vi "TreDadi.vi"() -> (1 "Dado_3":u32, 2 "Dado_2":u32, 3 "Dado_1":u32)   [LabVIEW 2013]
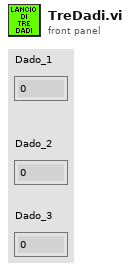
[diagram p1: front panel]
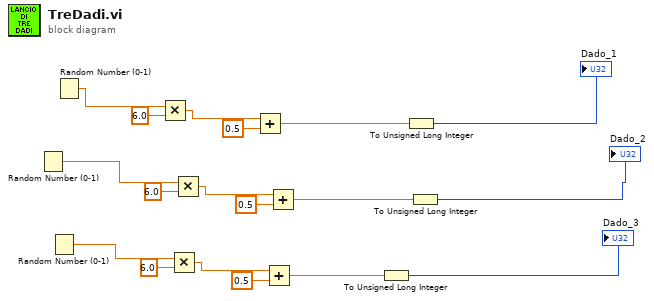
[diagram p0: block diagram]
diagram:
  n1 = Random Number (0-1)() -> (number: 0 to 1=w8:dbl)
  n2 = Random Number (0-1)() -> (number: 0 to 1=w7:dbl)
  n3 = Random Number (0-1)() -> (number: 0 to 1=w15:dbl)
  n4 = Multiply(x=w15, y=6.0) -> (x*y=w13:dbl)
  n5 = Multiply(x=w7, y=6.0) -> (x*y=w5:dbl)
  n6 = Multiply(x=w8, y=6.0) -> (x*y=w10:dbl)
  n7 = Add(x=w13, y=0.5) -> (x+y=w3:dbl)
  n8 = Add(x=w5, y=0.5) -> (x+y=w1:dbl)
  n9 = Add(x=w10, y=0.5) -> (x+y=w2:dbl)
  n10 = To Unsigned Long Integer(number=w1) -> (unsigned 32bit integer=→"Dado_3":u32)
  n11 = To Unsigned Long Integer(number=w3) -> (unsigned 32bit integer=→"Dado_1":u32)
  n12 = To Unsigned Long Integer(number=w2) -> (unsigned 32bit integer=→"Dado_2":u32)
